vi "PLC_OP30_Write.vi"(8 "error in (no error)":errorcluster, 11 "S7 Connection in":T1) -> (0 "error out":errorcluster, 3 "S7 Connection out":T1)   [LabVIEW 2017]
uses:
  <vilib>/DATA AHEAD/SP7/typedefs/S7 Connection.ctl
  <vilib>/DATA AHEAD/SP7/typedefs/PLC Type.ctl
  Global/DATA LOG.vi
  <vilib>/DATA AHEAD/SP7/functions/write/write Dint array.vi
  Global/Global 1.vi
  <vilib>/DATA AHEAD/SP7/functions/write/writeString.vi
  <vilib>/DATA AHEAD/SP7/SP7.lvlib
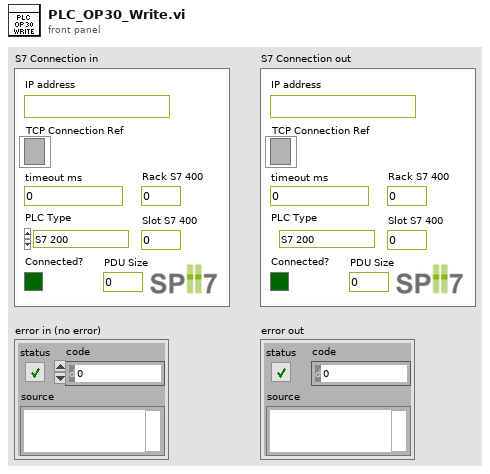
[diagram p1: front panel]
types:
  T1 = typedef "SP7.lvlib/S7 Connection.ctl" = cluster{"TCP Connection Ref":refnum<k5>, "IP address":string, "timeout ms":i32, "Connected?":bool, "PLC Type":T2, "Rack S7 400":u8, "Slot S7 400":u8, "PDU Size":u16, "connection semaphore":T3}
  T2 = typedef "SP7.lvlib/PLC Type.ctl" = enum16{"S7 200", "S7 300/400", "S7 1200", "S7 1500", "LOGO!8"}
  T3 = typedef "Semaphore RefNum" = refnum<k1>
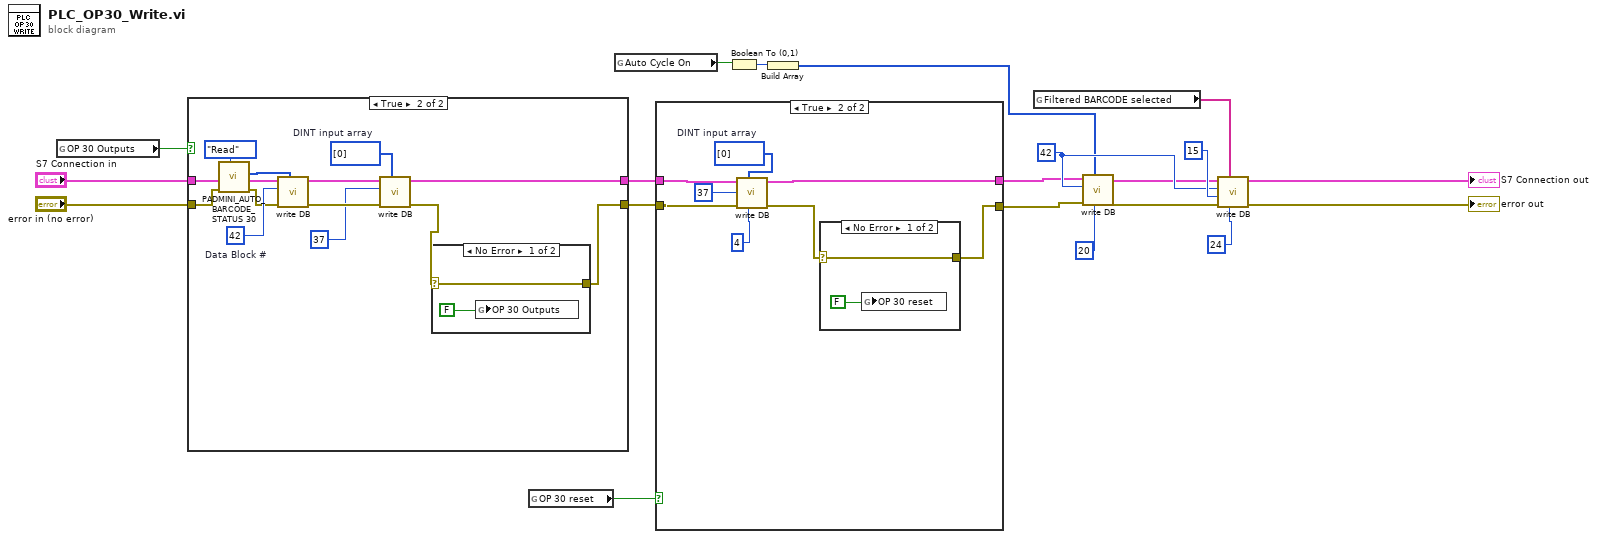
[diagram p0: block diagram]
diagram:
  w17 = u16 42 ("Data Block #")
  n1 = global read "DATA LOG.vi" "OP 30 Outputs"() -> (w6:bool)
  n2 = case shown="True" w6 {
    tunnel: "S7 Connection in" -> [w21 w34]
    tunnel: [w22 w23] -> w7
    tunnel: [w21 w28] -> w8
    tunnel: "error in (no error)" -> [w22 w31]
    frame False {
    }
    frame True {
      w26 = i32[] [0]  # DINT input array
      w35 = u16 42  # Data Block #
      n3 = call "PADMINI_AUTO_BARCODE_STATUS 30.vi"("Enum"=enum16{"Read", "Write"}."Read", "error in (no error)"=w31) -> ("error out"=w30:errorcluster, "O/P"=w32:i32[])  [unwired: 8 in]
      n4 = call-poly <vilib>:"write DB.vi"("DINT input array"=w32, "error in (no error)"=w30, "Data Block #"=w35, "S7 Connection in"=w34) -> ("error out"=w29:errorcluster, "S7 Connection out"=w27:T1)  [unwired: 4 in, 2 out]
      n5 = call-poly <vilib>:"write DB.vi"("DINT input array"=w26, "error in (no error)"=w29, "Data Block #"=u16 37, "S7 Connection in"=w27) -> ("error out"=w24:errorcluster, "S7 Connection out"=w28:T1)  [unwired: 4 in, 2 out]
      n6 = case shown="No Error" w24 {
        selector: w24 -> [w36 w38]
        tunnel: [w36 w38] -> w23
        frame No Error {
          n7 = global write "DATA LOG.vi" "OP 30 Outputs"(FALSE) -> ()
        }
        frame Error {
        }
      }
    }
  }
  n8 = global read "DATA LOG.vi" "OP 30 reset"() -> (w9:bool)
  n9 = global read "DATA LOG.vi" "Auto Cycle On"() -> (w3:bool)
  n10 = case shown="True" w9 {
    tunnel: w7 -> [w39 w48]
    tunnel: [w39 w41] -> w14
    tunnel: w8 -> [w40 w47]
    tunnel: [w40 w46] -> w12
    frame False {
    }
    frame True {
      w45 = i32[] [0]  # DINT input array
      n11 = call-poly <vilib>:"write DB.vi"("Item offset [byte]"=u16 4 ("Data Block #"), "DINT input array"=w45, "error in (no error)"=w48, "Data Block #"=u16 37, "S7 Connection in"=w47) -> ("error out"=w42:errorcluster, "S7 Connection out"=w46:T1)  [unwired: 3 in, 2 out]
      n12 = case shown="No Error" w42 {
        selector: w42 -> [w49 w51]
        tunnel: [w49 w51] -> w41
        frame No Error {
          n13 = global write "DATA LOG.vi" "OP 30 reset"(FALSE) -> ()
        }
        frame Error {
        }
      }
    }
  }
  n14 = Boolean To (0,1)(Boolean=w3) -> (0, 1=w2:i16)
  n15 = Build Array(w2) -> (w1:i16[])
  n16 = global read "Global 1.vi" "Filtered BARCODE selected"() -> (w20:string[])
  n17 = call-poly <vilib>:"write DB.vi"("Item offset [byte]"=u32 20, "DINT input array"=w1, "error in (no error)"=w14, "Data Block #"=w17, "S7 Connection in"=w12) -> ("error out"=w11:errorcluster, "S7 Connection out"=w10:T1)  [unwired: 3 in, 2 out]
  n18 = call-poly <vilib>:"write DB.vi"("Item offset [byte]"=u32 24, "Input STRINGS"=w20, "error in (no error)"=w11, "String length reserved in DB (default=254)"=u16 15, "Data Block #"=w17, "S7 Connection in"=w10) -> ("error out"=→"error out":errorcluster, "S7 Connection out"=→"S7 Connection out":T1)  [unwired: 2 in, 2 out]
